vi "IMS Stepper Control.vi"(2 "Point #":i32, 4 "Parameters":dbl[](array[numeric]) format="%.3e", 5 "Instrument Address":refnum<visa-resource-name>) -> (0 "Stop":bool, 1 "Data Out":dbl[](array[numeric]) format="%.2f")   [LabVIEW 2017]
doc: "Moves the stepper moter an appropriate amount based on the point number, step size and final position.\nScott Hannahs, NHMFL, March 1999"
uses:
  Serial Support VISA.llb/Serial Actions.ctl
panel:
  out "Starting Position":dbl format="%.2f"
  # "Motor Number"
  # "Step Size"
  # "Final Position"
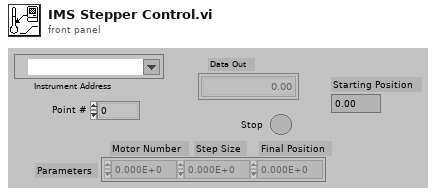
[diagram p1: front panel]
types:
  T1 = cluster{"Parameters[0]":dbl, "Parameters[1]":dbl, "Parameters[2]":dbl}
  T2 = typedef "Serial Actions.ctl" = enum16{"Init", "Break", "Clear Buffer", "Write", "Read", "N Bytes", "Lock", "Unlock", "Close"}
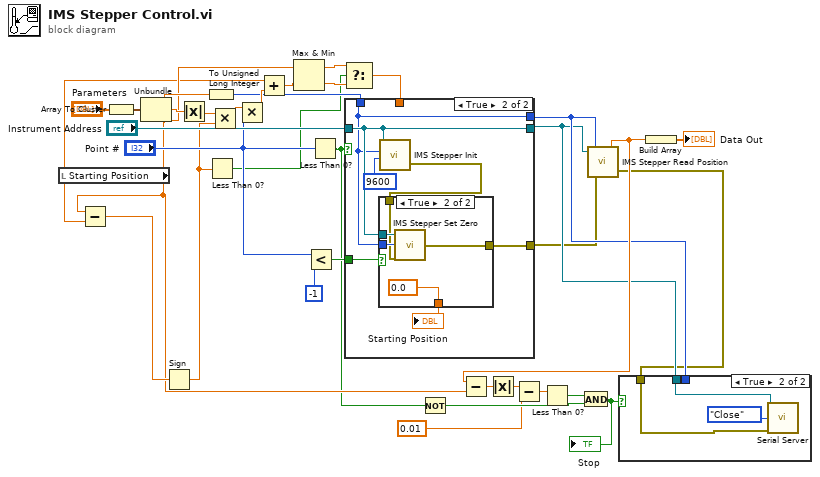
[diagram p0: block diagram]
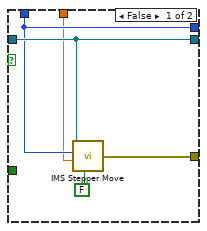
[diagram p3: hidden frame]
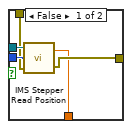
[diagram p4: hidden frame]
diagram:
  n1 = local read "Starting Position"() -> (w6:dbl)
  n2 = Array To Cluster(array="Parameters") -> (cluster=w34:T1)
  n3 = Unbundle(w34) -> ("Parameters[0]"=w31:dbl, "Parameters[1]"=w19:dbl, "Parameters[2]"=w12:dbl)
  n4 = Subtract(x=w12, y=w6) -> (x-y=w20:dbl)
  n5 = Sign(1:w20) -> (0:w11:dbl)
  n6 = Absolute Value(x=w19) -> (abs(x)=w17:dbl)
  n7 = To Unsigned Long Integer(number=w31) -> (unsigned 32bit integer=w25:u32)
  n8 = Less Than 0?(x=w11) -> (x < 0?=w10:bool)
  n9 = Multiply(x=w17, y=w11) -> (x*y=w18:dbl)
  n10 = Multiply(x=w18, y="Point #") -> (x*y=w33:dbl)
  n11 = Add(x=w6, y=w33) -> (x+y=w16:dbl)
  n12 = Max & Min(x=w12, y=w16) -> (max(x,y)=w14:dbl, min(x,y)=w13:dbl)
  n13 = Less?(x="Point #", y=-1) -> (x < y?=w22:bool)
  n14 = Less Than 0?(x="Point #") -> (x < 0?=w3:bool)
  n15 = Select(t=w14, s=w10, f=w13) -> (s? t:f=w15:dbl)
  n16 = case shown="True" w3 {
    tunnel: "Instrument Address" -> [w40 w43]
    tunnel: [w40 w43] -> w26
    tunnel: w25 -> [w39 w42]
    tunnel: [w39 w42] -> w27
    tunnel: [w38 w46] -> w7
    tunnel: w22 -> [_ w45]
    tunnel: w15 -> [w37 _]
    frame False {
      n17 = call "IMS Stepper Move.vi"("Instrument Address"=w40, "Motor Number"=w39, "Distance"=w37, "Mode"=FALSE) -> ("error out"=w38:errorcluster)  [unwired: 1 in]
    }
    frame True {
      n18 = call "IMS Stepper Init.vi"("Baud Rate"=u32 9600, "Motor Number"=w42, "Instrument Address"=w43) -> ("error out"=w41:errorcluster)  [unwired: 1 in, 1 out]
      n19 = case shown="True" w45 {
        tunnel: w42 -> [w52 w57]
        tunnel: w43 -> [w51 w56]
        tunnel: [w50 w55] -> w46
        tunnel: [w49 0.0] -> w44
        tunnel: w41 -> [w48 w53]
        frame False {
          n20 = call "IMS Stepper Read Position.vi"("error in (no error)"=w48, "Motor Number"=w52, "Instrument Address"=w51) -> ("error out"=w50:errorcluster, "Response"=w49:dbl)
        }
        frame True {
          n21 = call "IMS Stepper Set Zero.vi"("error in (no error)"=w53, "Motor Number"=w57, "Instrument Address"=w56) -> ("error out"=w55:errorcluster)
        }
      }
      "Starting Position" <- w44
    }
  }
  n22 = Not(x=w3) -> (.not. x?=w2:bool)
  n23 = call "IMS Stepper Read Position.vi"("error in (no error)"=w7, "Motor Number"=w27, "Instrument Address"=w26) -> ("error out"=w21:errorcluster, "Response"=w29:dbl)
  n24 = Subtract(x=w29, y=w12) -> (x-y=w28:dbl)
  n25 = Absolute Value(x=w28) -> (abs(x)=w9:dbl)
  n26 = Subtract(x=w9, y=0.01) -> (x-y=w8:dbl)
  n27 = Less Than 0?(x=w8) -> (x < 0?=w4:bool)
  n28 = And(x=w4, y=w2) -> (x .and. y?=w5:bool)
  "Stop" <- w5
  n29 = case shown="True" w5 {
    tunnel: w27 -> [_ _]
    tunnel: w26 -> [_ w59]
    tunnel: w21 -> [_ w58]
    frame False {
    }
    frame True {
      n30 = call "Serial Server.vi"("VISA Resource Name"=w59, "Action"=Serial_Actions."Close", "error in (no error)"=w58) -> ()  [unwired: 8 in, 5 out]
    }
  }
  n31 = Build Array(w29) -> (→"Data Out":dbl[])
